vi "Center VI on Monitor.vi"(4 "Close Reference (T)":bool=TRUE, 6 "VI Ref (calling VI)":refnum<vi>, 7 "Make Modal":bool, 8 "error in (no error)":errorcluster, 10 "Coords (Current Mouse)":T1={"Horizontal"=-1, "Vertical"=-1}, 11 "Window Mode (Center on Monitor)":enum16{"Center on Monitor", "Center on Mouse"}(ring)) -> (0 "error out":errorcluster)   [LabVIEW 2021, in "Panel Movement Center Maximize.lvlib"]
doc: "This VI will move a calling VIs front panel to the coordinates provided. If no coordinates are provided it moves to the current mouse position. This will by default move the window and center it on the monitor that the mouse is on. Other options are to center it under the mouse location, but keep it on the same monitor.\n\n-----\nHooovahh\n(Brian Hoover)"
uses:
  Panel Movement Center Maximize.lvlib
  <vilib>/Utility/miscctls.llb/LVPoint32TypeDef.ctl
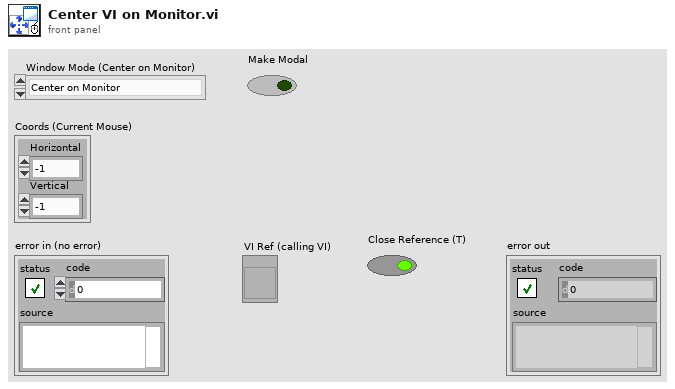
[diagram p1: front panel]
types:
  T1 = typedef "LVPoint32TypeDef.ctl" = cluster{"Horizontal":i32, "Vertical":i32}
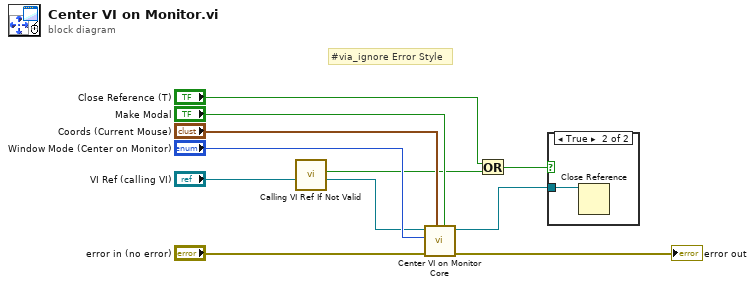
[diagram p0: block diagram]
diagram:
  # "#via_ignore Error Style"
  n1 = call "Calling VI Ref If Not Valid.vi"("VI Reference"="VI Ref (calling VI)") -> ("Valid VI Ref"=w7:refnum<vi>, "New Reference Opened"=w5:bool)  [unwired: 8 in, 1 out]
  n2 = call "Center VI on Monitor Core.vi"("Make Modal"="Make Modal", "Coords (Current Mouse)"="Coords (Current Mouse)", "error in (no error)"="error in (no error)", "Window Mode (Center on Monitor)"="Window Mode (Center on Monitor)", "VI Ref In"=w7) -> ("error out"=→"error out":errorcluster, "VI Ref Out"=w6:refnum<vi>)  [unwired: 5 in]
  n3 = Or(x="Close Reference (T)", y=w5) -> (x .or. y?=w3:bool)
  n4 = case shown="True" w3 {
    tunnel: w6 -> [_ w12]
    frame False {
    }
    frame True {
      n5 = Close Reference(reference=w12) -> ()  [unwired: 1 in, 1 out]
    }
  }
